vi "TTCM Config Range and Terminal Settings.vi"(0 "DAQmx Task In":refnum<k21>, 5 "Range and Terminal Settings":T1={"Global Settings"={"Min Temp (deg C)"=100.0, "Max Temp (deg C)"=0.0, "Thermocouple Type"=10072, "CJC Temp (deg C)"=25.0, "Enable Autozero"=FALSE, "Auto Zero Mode"=10230}, "Specific Channel Settings"=[]} {"Specific Channel Settings"."Thermocouple Type" items=["J"=10072, "K"=10073, "N"=10077, "R"=10082, "S"=10085, "T"=10086, "B"=10047, "E"=10055]; "Global Settings"."Auto Zero Mode" items=["None"=10230, "Once"=10244, "Every Sample"=10164]; "Global Settings"."Thermocouple Type" items=["J"=10072, "K"=10073, "N"=10077, "R"=10082, "S"=10085, "T"=10086, "B"=10047, "E"=10055]; "Global Settings"."CJC Temp (deg C)" format="%#.6f"; "Global Settings"."Min Temp (deg C)" format="%#.6f"; "Global Settings"."Max Temp (deg C)" format="%#.6f"}, 11 "error in (no error)":errorcluster) -> (4 "DAQmx Task Out":refnum<k21>, 15 "error out":errorcluster)   [LabVIEW 2021, in "DAQ_Temperature Thermocouple Measurement.lvlib"]
doc: "<B>Configure Range and Terminal Settings </B>\n<B>Global Settings </B>configures the range and terminal settings for all analog input temperature channels except the channels specified in the specific channel settings\n\n<B>Specific Channel Settings</B> the range and terminal settings for the physical analog input temperature channels. If the channels are specified in the list, the global settings will be applied."
uses:
  DAQ_Temperature Thermocouple Measurement.lvlib
  <resource>/objmgr/daqmx.rc
  Typedefs/Specific Channel Settings.ctl
  Typedefs/Range and Terminal Settings.ctl
panel:
  # "Physical Channel Name"
  # "Thermocouple Type"
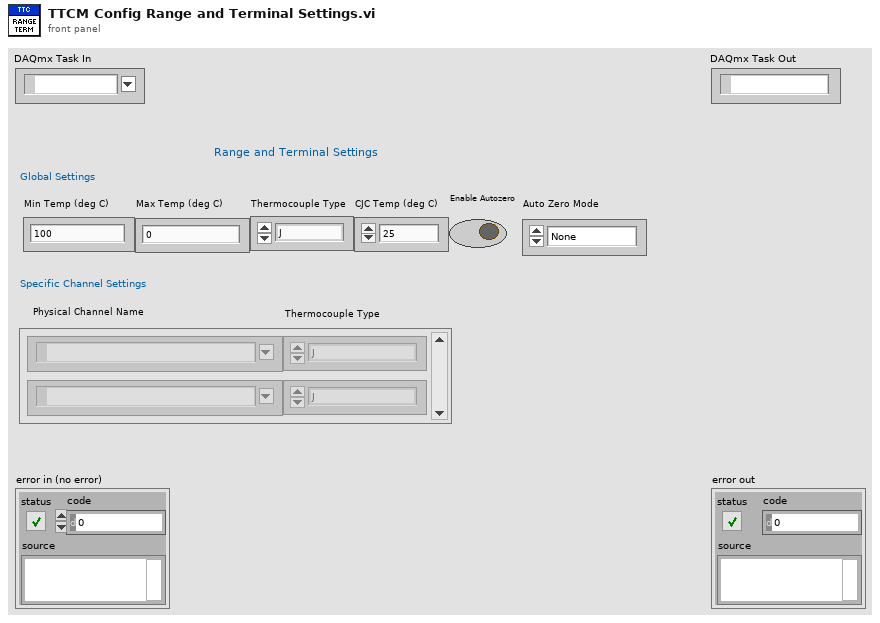
[diagram p1: front panel]
types:
  T1 = typedef "DAQ_Temperature Thermocouple Measurement.lvlib/Range and Terminal Settings.ctl" = cluster{"Global Settings":cluster{"Min Temp (deg C)":dbl, "Max Temp (deg C)":dbl, "Thermocouple Type":i32, "CJC Temp (deg C)":dbl, "Enable Autozero":bool, "Auto Zero Mode":i32}, "Specific Channel Settings":T2[]}
  T2 = typedef "DAQ_Temperature Thermocouple Measurement.lvlib/Specific Channel Settings.ctl" = cluster{"Physical Channel Name":tag, "Thermocouple Type":i32}
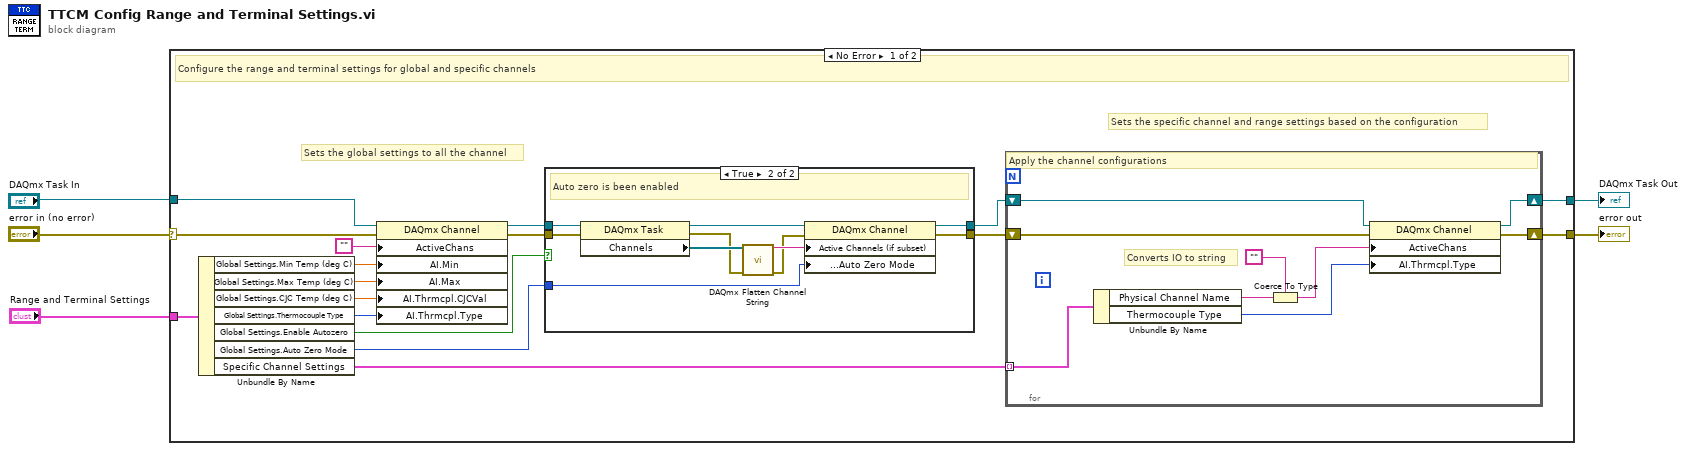
[diagram p0: block diagram]
diagram:
  n1 = case shown="No Error" "error in (no error)" {
    selector: "error in (no error)" -> [w18 w45]
    tunnel: "DAQmx Task In" -> [w19 w44]
    tunnel: "Range and Terminal Settings" -> [w17 _]
    tunnel: [w16 w44] -> w3
    tunnel: [w15 w45] -> w2
    frame No Error {
      # "Sets the specific channel and range settings based on the configuration"
      # "Sets the global settings to all the channel"
      # "Configure the range and terminal settings for global and specific channels"
      n2 = Unbundle By Name(w17) -> ("Global Settings.Min Temp (deg C)"=w21:dbl, "Global Settings.Max Temp (deg C)"=w22:dbl, "Global Settings.CJC Temp (deg C)"=w14:dbl, "Global Settings.Thermocouple Type"=w13:i32, "Global Settings.Enable Autozero"=w8:bool, "Global Settings.Auto Zero Mode"=w7:i32, "Specific Channel Settings"=w6:T2[])
      n3 = property class="DAQmx Channel"(reference=w19, error in=w18, "ActiveChans"="", "AI.Min"=w21, "AI.Max"=w22, "AI.Thrmcpl.CJCVal"=w14, "AI.Thrmcpl.Type"=w13) -> (reference out=w11:refnum<k21>, error out=w12:errorcluster)
      n4 = case shown="True" w8 {
        tunnel: w12 -> [w24 w29]
        tunnel: w11 -> [w23 w28]
        tunnel: [w24 w27] -> w10
        tunnel: [w23 w26] -> w9
        tunnel: w7 -> [_ w25]
        frame False {
          # "Auto zero disabled"
        }
        frame True {
          # "Auto zero is been enabled"
          n5 = property class="DAQmx Task"(reference=w28, error in=w29) -> (reference out=w34:refnum<k21>, error out=w31:errorcluster, "Channels"=w33:refnum<k21>[])
          n6 = call <vilib>:"DAQmx Flatten Channel String.vi"("names in"=w33, "error in"=w31) -> ("names out"=w32:string, "error out"=w30:errorcluster)  [unwired: 12 in]
          n7 = property class="DAQmx Channel"(reference=w34, error in=w30, "Active Channels (if subset)"=w32, "Analog Input:General Properties:Advanced:High Accuracy Settings:Auto Zero Mode"=w25) -> (reference out=w26:refnum<k21>, error out=w27:errorcluster)
        }
      }
      n8 = for {
        shift-right: [w41] -> w16
        shift-left: w9 -> [w42]
        shift-right: [w43] -> w15
        shift-left: w10 -> [w39]
        tunnel: w6 -> [w40] mode=indexing
        # "Converts IO to string"
        # "Apply the channel configurations"
        n9 = Unbundle By Name(w40) -> ("Physical Channel Name"=w37:tag, "Thermocouple Type"=w35:i32)
        n10 = Coerce To Type(0:w37, 1:"") -> (2:w36:string)
        n11 = property class="DAQmx Channel"(reference=w42, error in=w39, "ActiveChans"=w36, "AI.Thrmcpl.Type"=w35) -> (reference out=w41:refnum<k21>, error out=w43:errorcluster)
      }
    }
    frame Error {
      # "Error case - Do nothing"
    }
  }
  "DAQmx Task Out" <- w3
  "error out" <- w2
